vi "局部变量（滑动杆控制温度）.vi"() -> ()   [LabVIEW 2017]
panel:
  out "超高":bool
  out "初始值":dbl
  in  "滑动杆":dbl(slide) scale=0.0..50.0
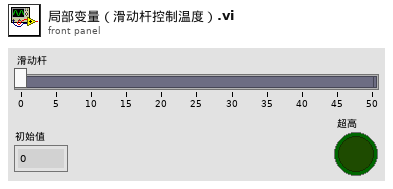
[diagram p1: front panel]
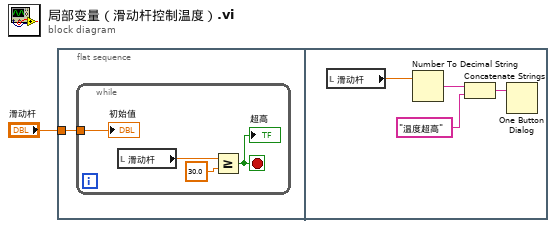
[diagram p0: block diagram]
diagram:
  n1 = flat-sequence {
    tunnel: "滑动杆" -> [w2]
    frame #0 {
      n2 = while {
        tunnel: w2 -> [w6]
        stop <- w3 stop-if-true
        n3 = local read "滑动杆"() -> (w5:dbl)
        n4 = Greater Or Equal?(x=w5, y=30.0) -> (x >= y?=w3:bool)
        "超高" <- w3
        "初始值" <- w6
      }
    }
    frame #1 {
      n5 = local read "滑动杆"() -> (w10:dbl)
      n6 = Number To Decimal String(number=w10) -> (decimal integer string=w8:string)  [unwired: 1 in]
      n7 = Concatenate Strings(w8, "温度超高") -> (w9:string)
      n8 = One Button Dialog(message=w9) -> ()  [unwired: 1 in, 1 out]
    }
  }
